vi "GetFileHexapodFTP.vi"(3 "error in (no error)":errorcluster caption="entrée d'erreur (pas d'erreur)", 4 "HexapodFileName":string="tete.txt", 5 "NomProjet":string) -> (0 "error out":errorcluster caption="sortie d'erreur", 2 "NomProjetOut":string)   [LabVIEW 2015]
uses:
  DefDeType/WhichPath.ctl
  <vilib>/FTP/NI_FTP.lvlib
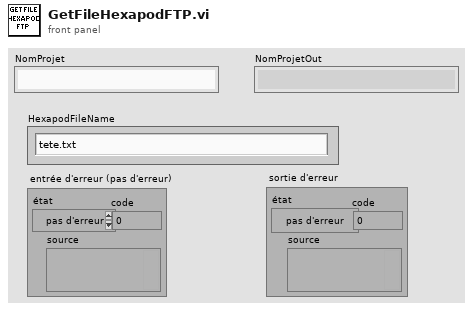
[diagram p1: front panel]
types:
  T1 = typedef "WhichPath.ctl" = enum16{"DossierProjet", "Config", "Meas", "MeasSuitCase", "MeasOnBoard", "MeasQualisys", "MeasTDMS", "MeasHexapode", "MeasNortek", "Fig", "Res"}
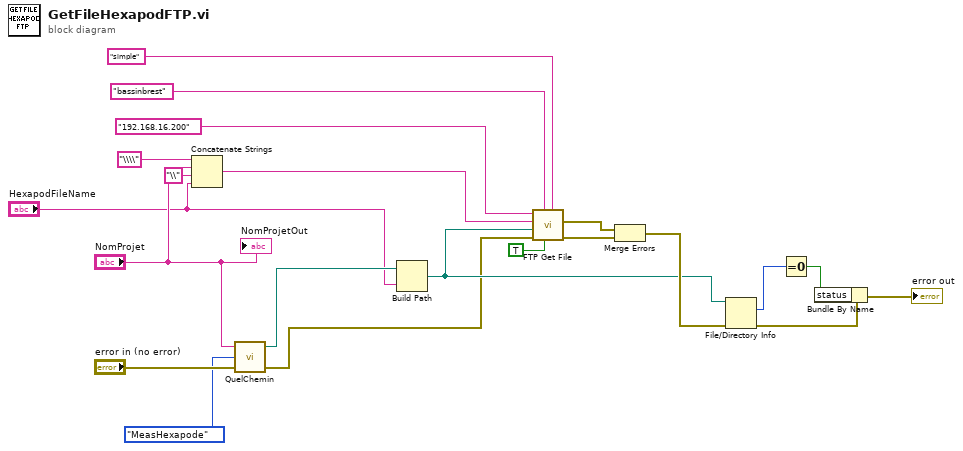
[diagram p0: block diagram]
diagram:
  n1 = Concatenate Strings("\\\\" ("chaîne"), "NomProjet", "\\" ("string"), "HexapodFileName") -> (w14:string)
  n2 = call "QuelChemin.vi"("Entrée d'erreur"="error in (no error)", "WhichPath?"=WhichPath."MeasHexapode", "NomProjet"="NomProjet") -> ("Sortie d'erreur"=w6:errorcluster, "SurDisqueLocal"=w3:path)  [unwired: 1 out]
  n3 = Build Path(base path=w3, name or relative path="HexapodFileName") -> (appended path=w12:path)
  n4 = call <vilib>:"FTP Get File.vi"("password"="simple", "binary (F)"=TRUE, "user"="bassinbrest", "error in (no error)"=w6, "local path"=w12, "remote path"=w14, "host"="192.168.16.200") -> ("error out"=w16:errorcluster, "file error"=w17:errorcluster)  [unwired: 3 in]
  n5 = Merge Errors(w17, w16) -> (w13:errorcluster)
  n6 = File/Directory Info(path=w12, error in=w13) -> (size=w11:i64, error out=w8:errorcluster)  [unwired: 5 out]
  n7 = Equal To 0?(x=w11) -> (x = 0?=w10:bool)
  n8 = Bundle By Name(cluster=w8, "status"=w10) -> (→"error out":errorcluster)
  "NomProjetOut" <- "NomProjet"
